vi "Process.vi"(8 "error in":errorcluster, 11 "RemoteControl":refnum<class "RemoteControl.lvclass">) -> (0 "error out":errorcluster, 3 "RemoteControl out":refnum<class "RemoteControl.lvclass">)   [LabVIEW 2016, in "RemoteControl.lvclass"]
doc: "---------------------------------------------------------------\nJKI State Machine Objects™\nhttp://jki.net/state-machine-objects/\nCopyright (C) 2005-2015, JKI <info@jki.net>\nALL RIGHTS RESERVED"
uses:
  RemoteControl.lvclass
  C:/Program Files (x86)/National Instruments/LabVIEW 2016/vi.lib/JKI/JKI SMO/SMO/SMO.lvclass
  <vilib>/NI/STM/SubVIs/MetaDataElement.ctl
  <vilib>/JKI/JKI SMO/SMO/Typedefs/Parent Call--Enum.ctl
  Typedefs/Remote-SMO-Commands-Enum.ctl
  Typedefs/PrivateEvents--RemoteControl.setAllowedRemoteAddress.ctl
  Typedefs/PrivateEvents--RemoteControl.setResults.ctl
  Typedefs/PrivateEvents--RemoteControl.setAO.ctl
  Typedefs/PrivateEvents--RemoteControl.setAI.ctl
  Typedefs/PrivateEvents--RemoteControl.setTrigger.ctl
  Typedefs/REF-cluster.ctl
  Typedefs/REF_f-array.ctl
  Typedefs/REF_phi-array.ctl
  Typedefs/AO-cluster.ctl
  Typedefs/AO_Amp-array.ctl
  Typedefs/AO_DC-array.ctl
  Typedefs/AO_f-array.ctl
  Typedefs/AO_phi-array.ctl
  Typedefs/Function-array.ctl
  Typedefs/Function-enum.ctl
  Typedefs/PrivateEvents--RemoteControl.setIVmode.ctl
  RemoteControl.lvclass/RemoteControl.ctl
  <vilib>/NI/STM/TCP/TCP Read Options.ctl
  Typedefs/PublicEvents--RemoteControl.configAO.ctl
  Typedefs/PublicEvents--RemoteControl.configREF.ctl
  Typedefs/PublicEvents--RemoteControl.configIVmode.ctl
  Typedefs/PublicEvents--RemoteControl.configRemote.ctl
  Typedefs/PublicEvents--RemoteControl.configReset.ctl
  Typedefs/PublicEvents--RemoteControl.assertTrigger.ctl
  <vilib>/NI/STM/TCP/Write Meta Data (TCP Ref).vi
  <vilib>/NI/STM/TCP/Get Connection Reference (TCP).vi
  <userlib>/_OpenG.lib/error/error.llb/Filter Error Codes (Array)__ogtk.vi
  <vilib>/NI/STM/TCP/Write Meta Data (TCP Clst).vi
  <vilib>/NI/STM/TCP/Read Message (TCP).vi
  <vilib>/NI/STM/TCP/Write Message (TCP).vi
  <vilib>/JKI/JKI SMO/SMO/SMO.lvclass
  <vilib>/NI/STM/NI STM.lvlib
  <vilib>/addons/_JKI.lib/Serialization/JSON/JKI JSON Serialization.lvlib
panel:
  out "states":string
  out "commands":string
  out "data string":string
  out "command":T1
  # "For instructions on how to use the JKI State Machine Objects, examples and video tutorials, visit:\nhttp://jki.net/state-machine-objects/\n\nJKI State Machine Objects™\nhttp://jki.net/state-machine-objects/\nCopyright (C) 2005-2015, JKI <info@jki.net>\nALL RIGHTS RESERVED"
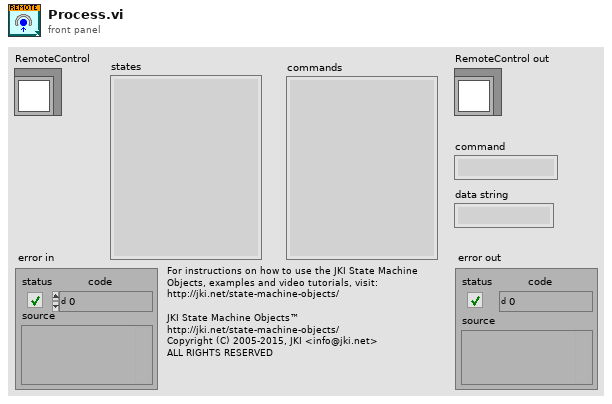
[diagram p1: front panel]
types:
  T1 = typedef "NI STM.lvlib/MetaDataElement.ctl" = string
  T2 = typedef "RemoteControl.lvclass/Remote-SMO-Commands-Enum.ctl" = enum16{"configAO", "configREF", "configIVmode", "configRemote", "configReset", "assertTrigger", "getAO", "getAI", "getResults", "getTrigger", "getIVmode", "getAOconfig", "getREFconfig", "ACK", "UNK", "CLOSE"}
  T3 = typedef "SMO.lvclass/Parent Call--Enum.ctl" = enum16{"Allows parent to run", "Does not request parent to run"}
  T4 = enum32{"invalid app kind", "Development System", "Run Time System", "Student Edition", "Embedded LabVIEW", "Evaluation", "Custom"}
  T5 = enum32{"Invalid", "Standard", "Closed", "Hidden", "Minimized", "Maximized"}
  T6 = enum32{"Bad", "Idle", "Run top level", "Running"}
  T7 = typedef "NI STM.lvlib/TCP Read Options.ctl" = cluster{"ignore timeout error":bool, "timeout ms (1000)":i32}
  T8 = typedef "RemoteControl.lvclass/PrivateEvents--RemoteControl.setAllowedRemoteAddress.ctl" = string
  T9 = typedef "NI STM.lvlib/TCP Connection Info.ctl" = cluster{"connection ID":refnum<k5>, "meta data":T1[]}
  T10 = typedef "RemoteControl.lvclass/PrivateEvents--RemoteControl.setAO.ctl" = waveform(dbl)[]
  T11 = typedef "RemoteControl.lvclass/PrivateEvents--RemoteControl.setAI.ctl" = waveform(dbl)[]
  T12 = typedef "RemoteControl.lvclass/PrivateEvents--RemoteControl.setResults.ctl" = dbl[][]
  T13 = typedef "RemoteControl.lvclass/PrivateEvents--RemoteControl.setTrigger.ctl" = bool
  T14 = typedef "AO-cluster.ctl" = cluster{"AO amp (V)":T15, "AO DC (V)":T16, "AO f (Hz)":T17, "AO phi (deg)":T18, "function":T19}
  T15 = typedef "AO_Amp-array.ctl" = dbl[]
  T16 = typedef "AO_DC-array.ctl" = dbl[]
  T17 = typedef "AO_f-array.ctl" = dbl[]
  T18 = typedef "AO_phi-array.ctl" = dbl[]
  T19 = typedef "Function-array.ctl" = T20[]
  T20 = typedef "Function-enum.ctl" = enum16{"Sine Wave", "Triangle Wave", "Square Wave", "Sawtooth Wave"}
  T21 = typedef "REF-cluster.ctl" = cluster{"REF f (Hz)":T22, "REF phi (deg)":T23}
  T22 = typedef "REF_f-array.ctl" = dbl[]
  T23 = typedef "REF_phi-array.ctl" = dbl[]
  T24 = typedef "RemoteControl.lvclass/PrivateEvents--RemoteControl.setIVmode.ctl" = bool
  T25 = cluster{"Core":cluster{"Current VI Reference":refnum<vi>, "Close Panel on Exit?":bool, "error":errorcluster}, "Self Reference":refnum<class "RemoteControl.lvclass">, "STP info":cluster{"address":string, "port":u16, "STP connection info":T9}, "remote address":string, "remote port":u16, "data string":string, "command":T1, "AllowedRemoteAddress":T8, "LocalAddress":string, "setAO":T10, "setAI":T11, "setResults":T12, "setTrigger":T13, "Channels: AO":T14, "Channels: Lockin":T21, "setIVmode":T24}
  T26 = cluster{"Current VI Reference":refnum<vi>, "Close Panel on Exit?":bool, "error":errorcluster}
  T27 = cluster{"address":string, "port":u16, "STP connection info":T9}
  T28 = typedef "SMO.lvclass/Protected Events.ctl" = cluster{"StopProcesses":refnum<user-event>, "AbortProcesses":refnum<user-event>, "Config Changed":refnum<user-event>, "Dependency":refnum<user-event>}
  T29 = typedef "RemoteControl.lvclass/PrivateEvents--Cluster.ctl" = cluster{"setAllowedRemoteAddress":refnum<user-event>, "setAO":refnum<user-event>, "setAI":refnum<user-event>, "setResults":refnum<user-event>, "setTrigger":refnum<user-event>, "setAOconfig":refnum<user-event>, "setREFconfig":refnum<user-event>, "setReset":refnum<user-event>, "setIVmode":refnum<user-event>}
  T30 = typedef "RemoteControl.lvclass/PublicEvents--RemoteControl.configAO.ctl" = cluster{"Channels: AO":T14}
  T31 = typedef "RemoteControl.lvclass/PublicEvents--RemoteControl.configREF.ctl" = cluster{"Channels: Lockin":T21}
  T32 = typedef "RemoteControl.lvclass/PublicEvents--RemoteControl.configIVmode.ctl" = bool
  T33 = typedef "RemoteControl.lvclass/PublicEvents--RemoteControl.configRemote.ctl" = bool
  T34 = typedef "RemoteControl.lvclass/PublicEvents--RemoteControl.configReset.ctl" = bool
  T35 = typedef "RemoteControl.lvclass/PublicEvents--RemoteControl.assertTrigger.ctl" = bool
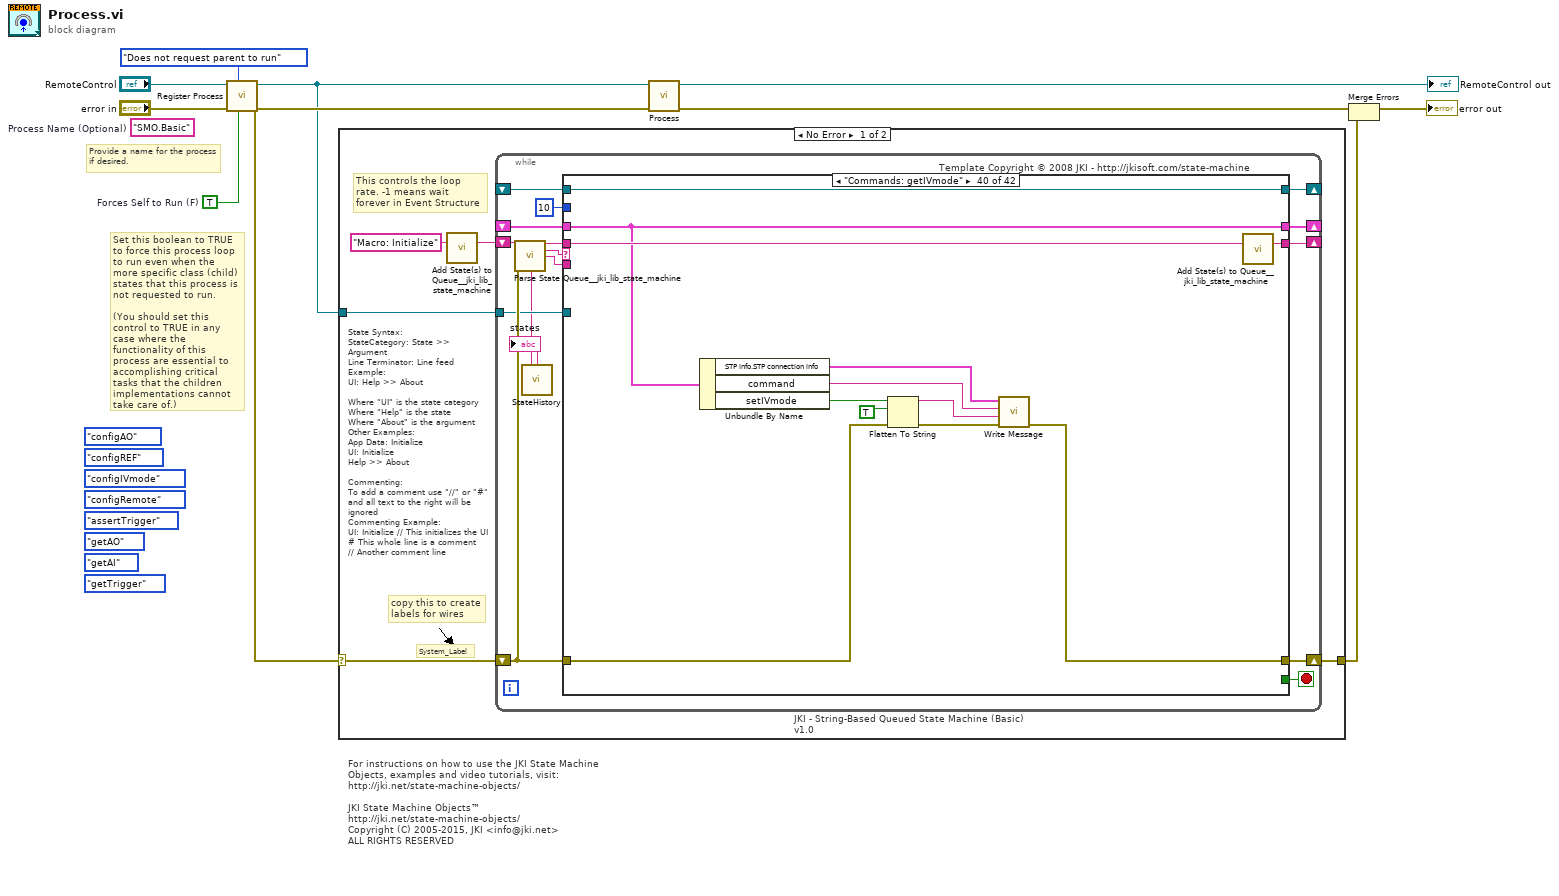
[diagram p0: block diagram]
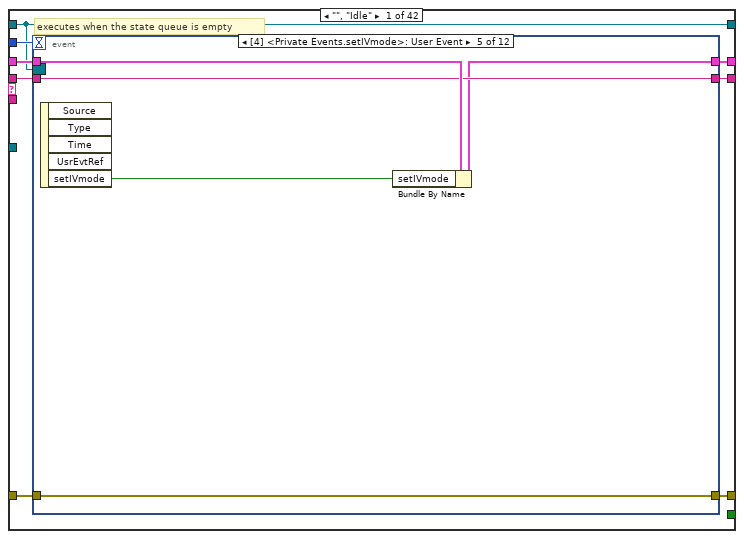
[diagram p2: hidden frame]
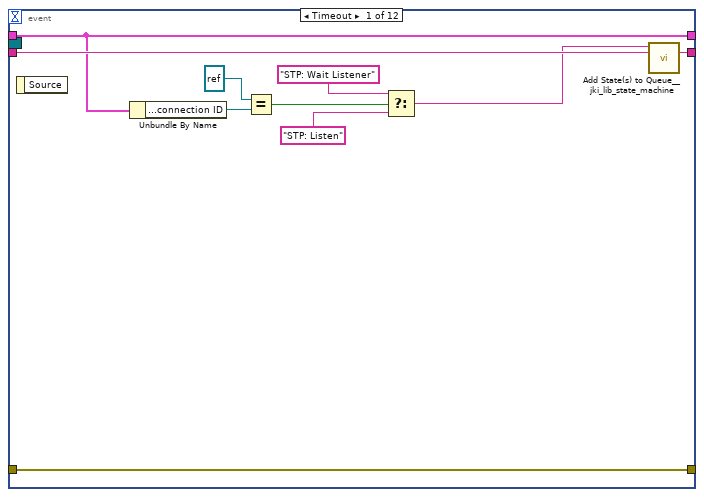
[diagram p3: hidden frame]
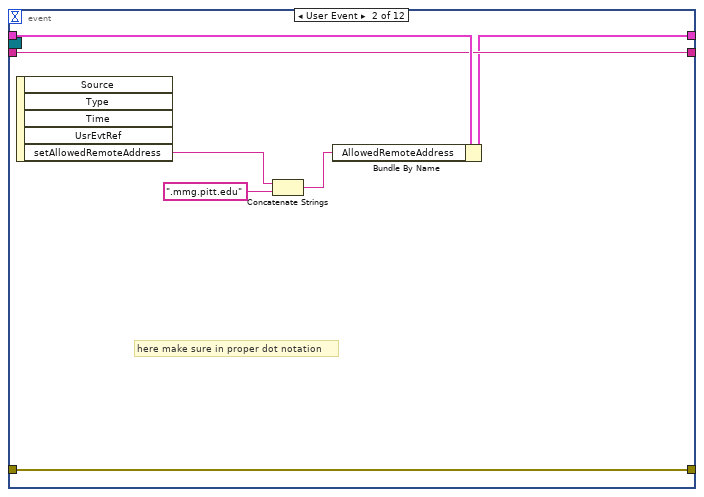
[diagram p4: hidden frame]
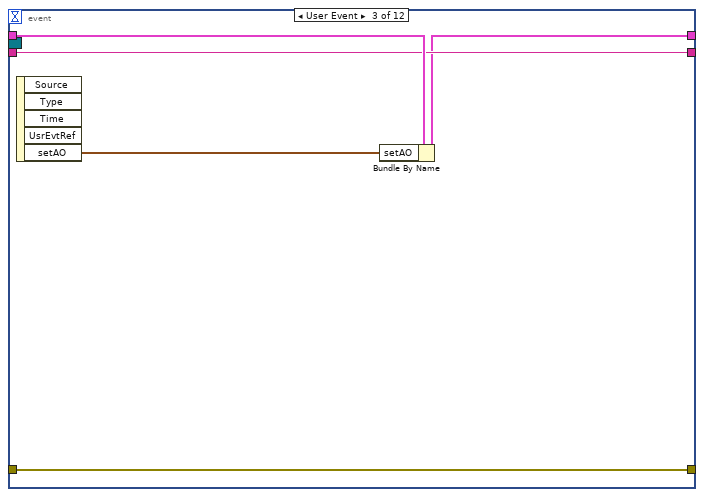
[diagram p5: hidden frame]
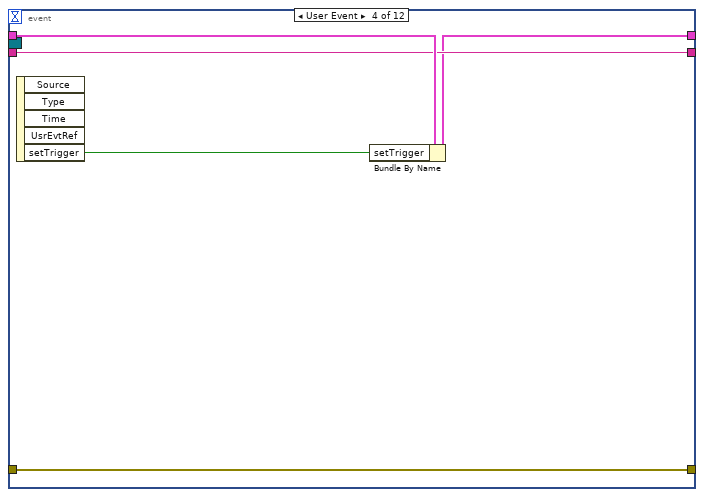
[diagram p6: hidden frame]
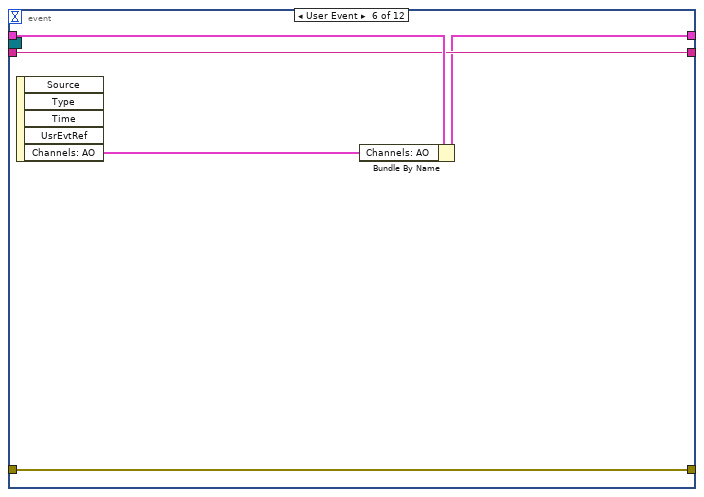
[diagram p7: hidden frame]
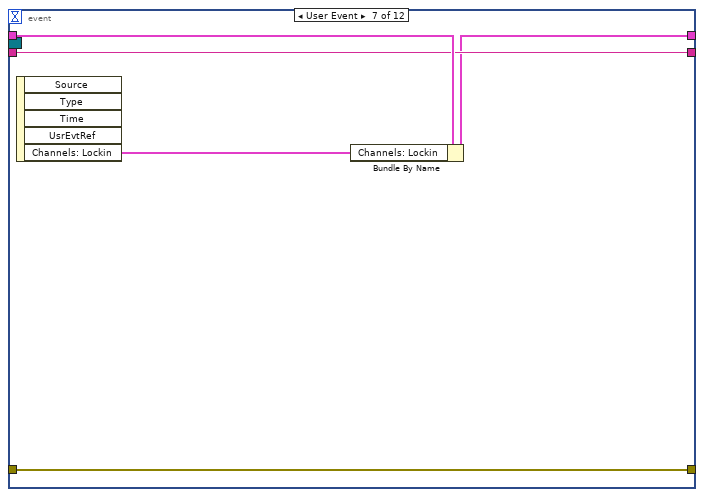
[diagram p8: hidden frame]
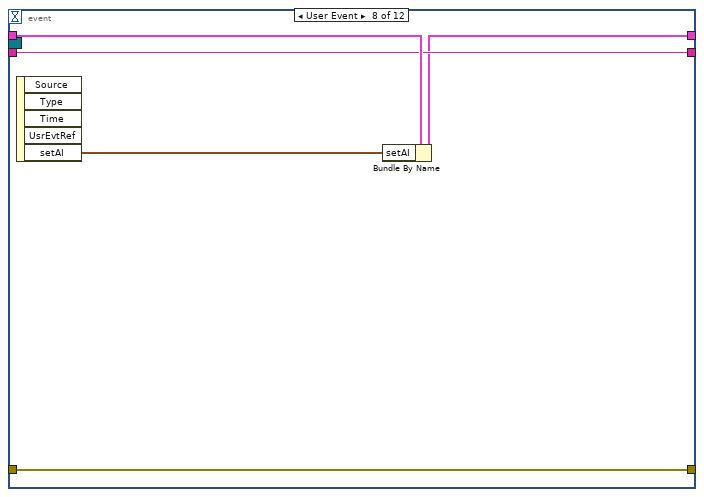
[diagram p9: hidden frame]
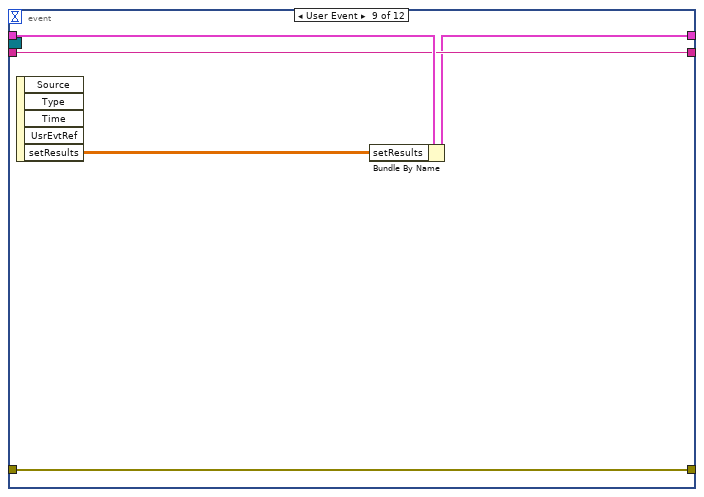
[diagram p10: hidden frame]
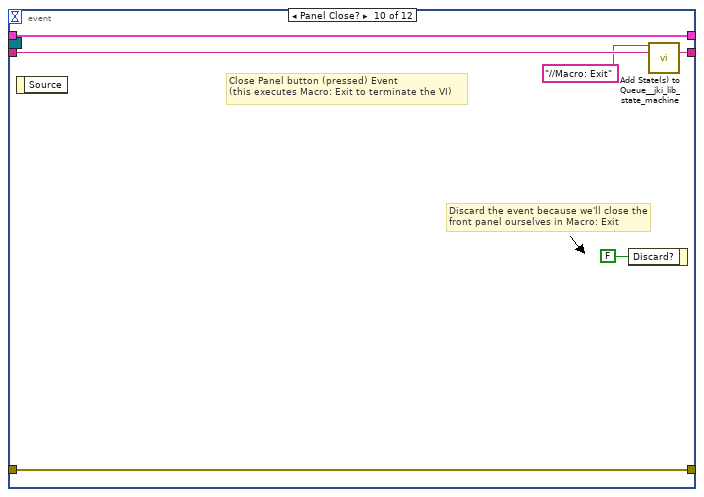
[diagram p11: hidden frame]
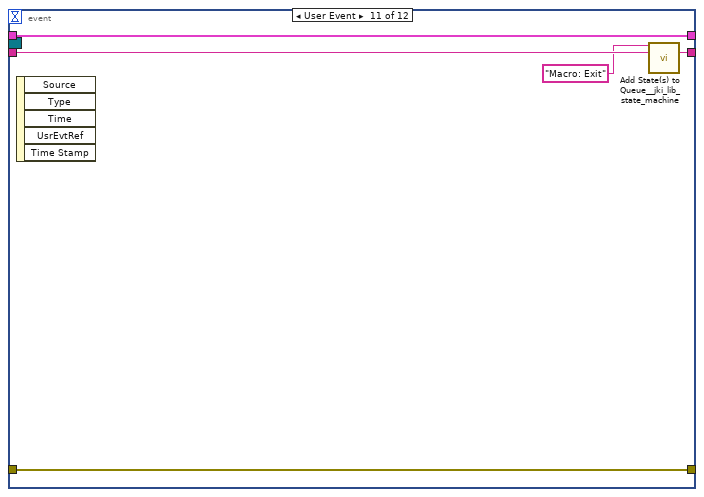
[diagram p12: hidden frame]
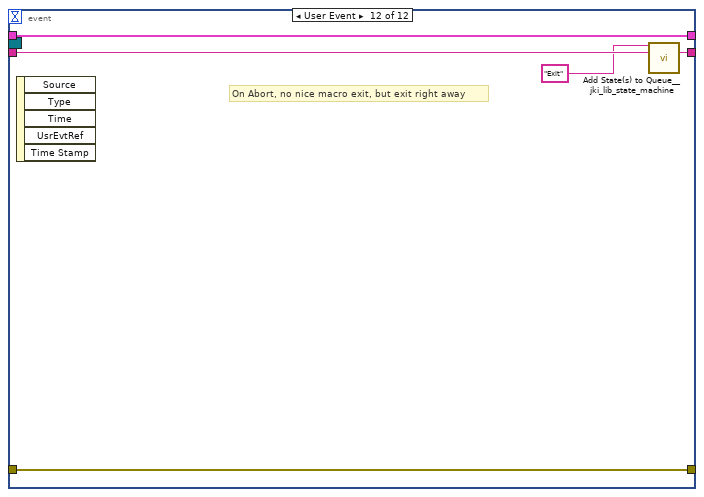
[diagram p13: hidden frame]
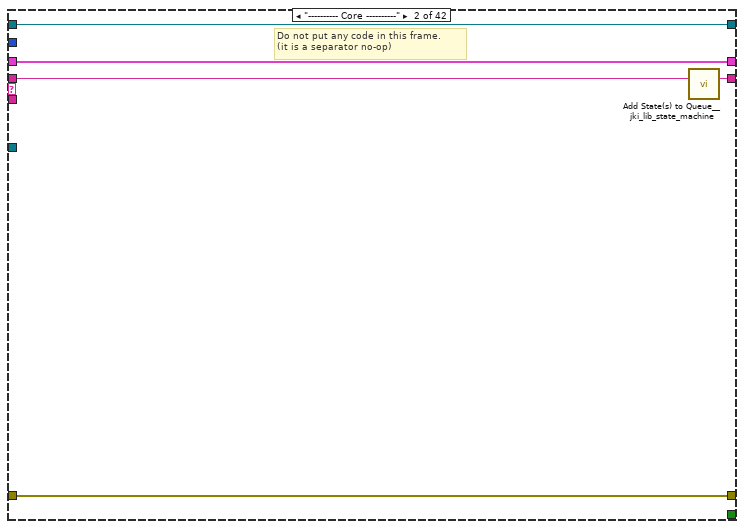
[diagram p14: hidden frame]
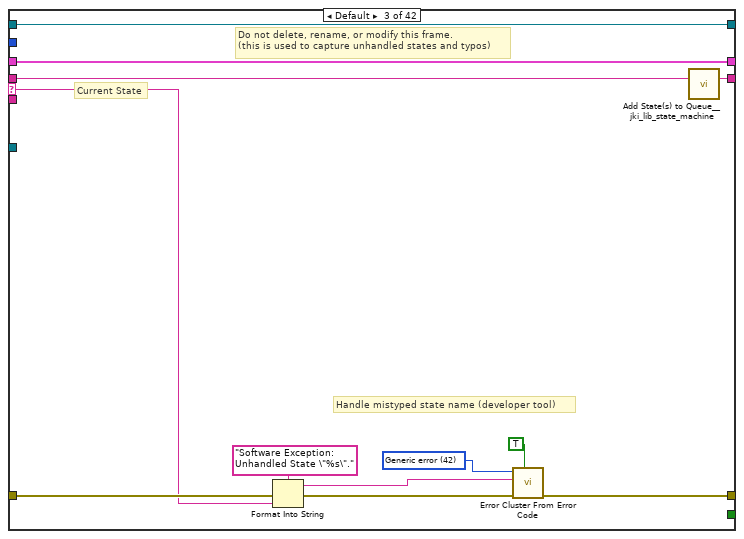
[diagram p15: hidden frame]
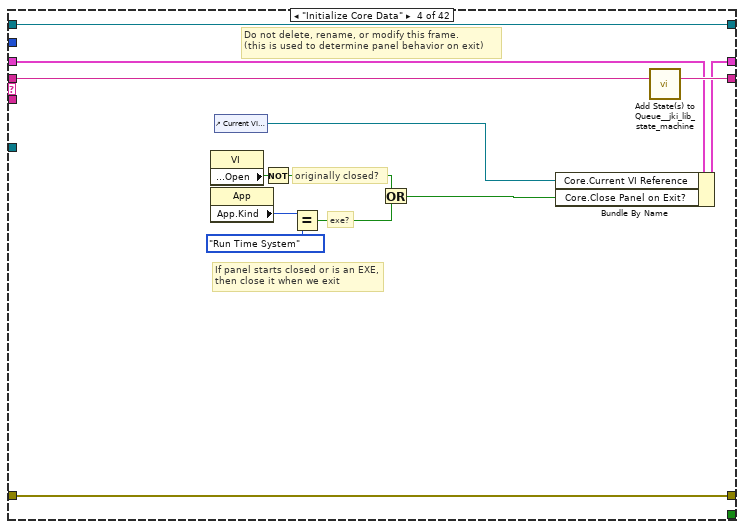
[diagram p16: hidden frame]
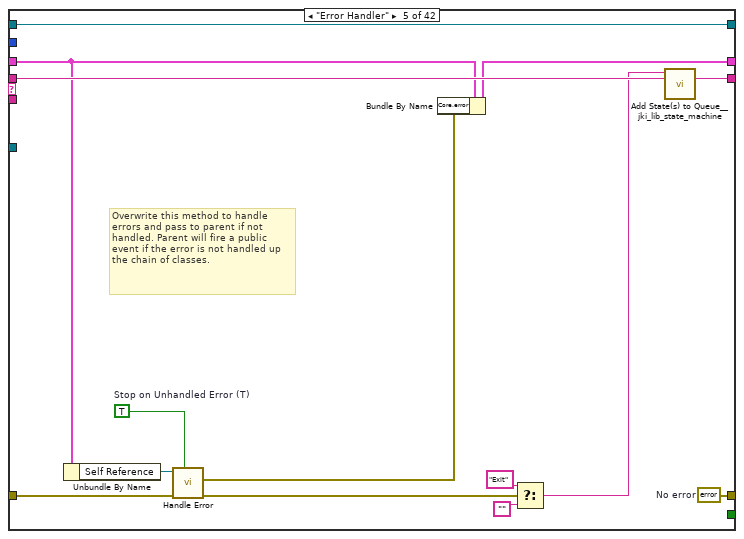
[diagram p17: hidden frame]
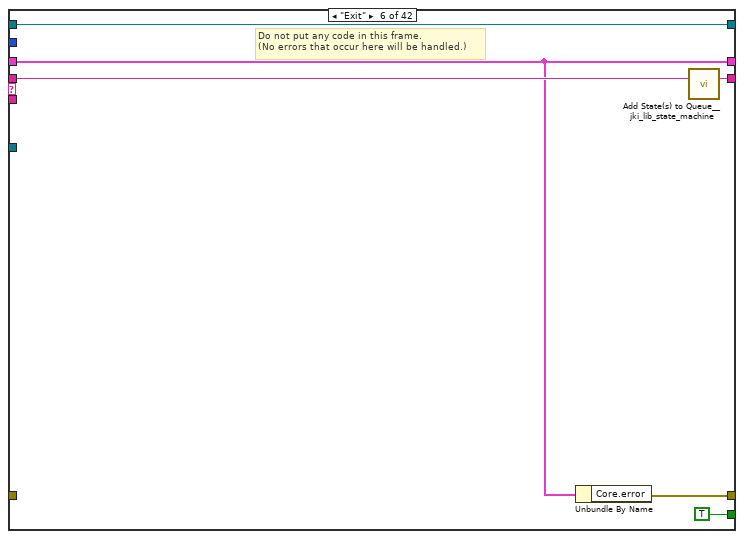
[diagram p18: hidden frame]
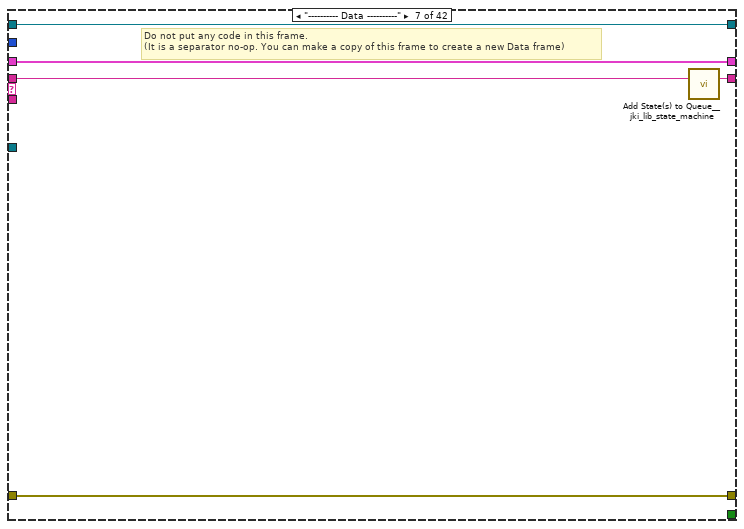
[diagram p19: hidden frame]
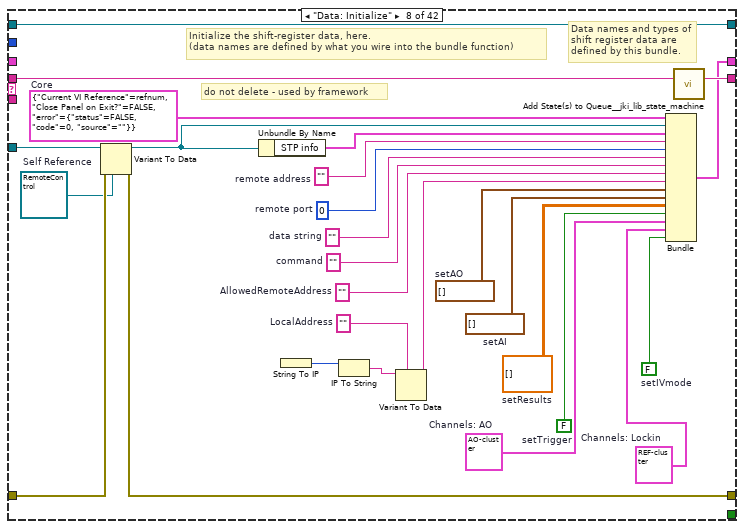
[diagram p20: hidden frame]
diagram:
  (unwired) Remote-SMO-Commands-Enum."getTrigger" ("Enum")
  (unwired) Remote-SMO-Commands-Enum."getAI" ("Enum")
  (unwired) Remote-SMO-Commands-Enum."getAO" ("Enum")
  (unwired) Remote-SMO-Commands-Enum."assertTrigger" ("Enum")
  (unwired) Remote-SMO-Commands-Enum."configRemote" ("Enum")
  (unwired) Remote-SMO-Commands-Enum."configIVmode" ("Enum")
  (unwired) Remote-SMO-Commands-Enum."configREF" ("Enum")
  (unwired) Remote-SMO-Commands-Enum."configAO" ("Enum")
  w1 = TRUE  # Forces Self to Run (F)
  (unwired) "SMO.Basic"  # Process Name (Optional)
  # "Provide a name for the process\nif desired."
  # "Set this boolean to TRUE to force this process loop to run even when the more specific class (child) states that this process is not requested to run.\n\n(You should set this control to TRUE in any case where the functionality of this process are essential to accomplishing critical tasks that the children implementations cannot take care of.)"
  # "For instructions on how to use the JKI State Machine Objects, examples and video tutorials, visit:\nhttp://jki.net/state-machine-objects/\n\nJKI State Machine Objects™\nhttp://jki.net/state-machine-objects/\nCopyright (C) 2005-2015, JKI <info@jki.net>\nALL RIGHTS RESERVED"
  n1 = call <vilib>:"Register Process.vi"("Forces Self to Run (F)"=w1, "Parent Call"=Parent_Call--Enum."Does not request parent to run", "error in (no error)"="error in", "SMO"="RemoteControl") -> ("error out"=w7:errorcluster, "SMO out"=w6:refnum<class "RemoteControl.lvclass">)  [unwired: 6 in]
  n2 = case shown="No Error" w7 {
    selector: w7 -> [w12 w652]
    tunnel: w6 -> [w13 _]
    tunnel: [w11 w652] -> w3
    frame No Error {
      # "State Syntax:\nStateCategory: State >> Argument\nLine Terminator: Line feed\nExample:\nUI: Help >> About\n\nWhere \"UI\" is the state category\nWhere \"Help\" is the state\nWhere \"About\" is the argument\nOther Examples:\nApp Data: Initialize\nUI: Initialize\nHelp >> About\n\nCommenting:\nTo add a comment use \"//\" or \"#\" and all text to the right will be ignored\nCommenting Example:\nUI: Initialize // This initializes the UI\n# This whole line is a comment\n// Another comment line"
      # "copy this to create labels for wires"
      # "This controls the loop rate. -1 means wait forever in Event Structure"
      # "System_Label"
      n3 = call <vilib>:"Add State(s) to Queue__jki_lib_state_machine.vi"("State(s) in (\"\")"="Macro: Initialize") -> ("States Out"=w15:string)  [unwired: 14 in]
      n4 = while "JKI - String-Based Queued State Machine (Basic) v1.0" {
        shift-right: [w24] -> _
        shift-left: _ -> [w23]
        shift-right: [w27] -> w11
        shift-left: w12 -> [w21]
        shift-right: [w26] -> _
        shift-left: w15 -> [w17]
        tunnel: w13 -> [w20]
        shift-right: [w19] -> _
        shift-left: _ -> [w18]
        stop <- w25 stop-if-true
        # "Template Copyright © 2008 JKI - http://jkisoft.com/state-machine"
        n5 = call <vilib>:"Parse State Queue__jki_lib_state_machine.vi"("State Queue"=w17, "Error In (no error)"=w21) -> ("Remaining States"=w29:string, "Current State"=w30:string, "Arguments"=w28:string)  [unwired: 11 in]
        n6 = call "StateHistory.vi"("Current State in"=w17) -> ("delimited string"=→"states":string)  [unwired: 9 in, 1 out]
        n7 = case shown="\"Commands: getIVmode\"" w30 {
          selector: w30 -> [_ _ w113 _ _ _ _ _ _ _ _ _ _ _ _ _ _ _ _ _ _ _ _ _ _ _ _ _ _ _ _ _ _ _ _ _ _ _ _ _ _ _]
          tunnel: w29 -> [w38 w111 w117 w136 w150 w156 w161 w188 w195 w200 w205 w212 w228 w260 w274 w288 w293 w304 w309 w322 w328 w333 w353 w391 w408 w450 w468 w480 w485 w500 w515 w528 w541 w554 w567 w579 w591 w603 w615 w627 w639 w651]
          tunnel: w28 -> [_ _ _ _ _ _ _ _ _ _ _ w206 w222 _ _ _ _ _ _ _ _ _ _ _ _ _ _ _ _ _ _ _ _ _ _ _ _ _ _ _ _ _]
          tunnel: w23 -> [w36 w108 w115 w127 w144 w152 w158 _ w190 w197 w203 w210 w224 w257 w270 w279 w290 w301 w306 w320 w326 w331 w342 w388 w405 w437 w455 w472 w483 w493 w507 w516 w537 w551 w564 w576 w587 w599 w611 w623 w635 w647]
          tunnel: [w35 w109 w119 w133 w145 w151 w159 w184 w191 w198 w202 w207 w225 w258 w272 w286 w291 w295 w307 w315 w324 w329 w348 w384 w394 w444 w462 w469 w481 w491 w505 w517 w536 w543 w555 w570 w581 w593 w605 w617 w629 w641] -> w27
          tunnel: w21 -> [w34 w109 w118 w133 w146 _ w159 w185 w192 w198 w202 w208 w226 w258 w272 w286 w291 w296 w307 w316 w324 w329 w349 w385 w402 w445 w463 w475 w481 w492 w506 w520 w533 w548 w561 w571 w582 w594 w606 w618 w630 w642]
          tunnel: [w37 w110 w116 w135 w149 w155 w160 w187 w194 w199 w204 w211 w227 w259 w273 w287 w292 w303 w308 w321 w327 w332 w352 w390 w407 w449 w467 w479 w484 w499 w514 w527 w540 w553 w566 w578 w590 w602 w614 w626 w638 w650] -> w26
          tunnel: [_ _ _ _ _ TRUE _ _ _ _ _ _ _ _ _ _ _ _ _ _ _ _ _ _ _ _ _ _ _ _ _ _ _ _ _ _ _ _ _ _ _ _] -> w25
          tunnel: [w33 w108 w115 w134 w143 w152 w158 w186 w190 w197 w203 w210 w224 w257 w270 w279 w290 w301 w306 w320 w326 w331 w347 w387 w404 w436 w454 w471 w483 w493 w507 w516 w537 w551 w564 w576 w587 w599 w611 w623 w635 w647] -> w24
          tunnel: 10 ("Timeout") -> [w32 _ _ _ _ _ _ _ _ _ _ _ _ _ _ _ _ _ _ _ _ _ _ _ _ _ _ _ _ _ _ _ _ _ _ _ _ _ _ _ _ _]
          tunnel: w20 -> [_ _ _ _ _ _ _ w182 _ _ _ _ _ _ _ _ _ _ _ _ _ _ _ _ _ _ _ _ _ _ _ _ _ _ _ _ _ _ _ _ _ _]
          tunnel: [w31 w107 w112 w124 w148 w153 w157 w181 w189 w196 w201 w209 w221 w256 w271 w280 w289 w302 w305 w319 w325 w330 w351 w389 w406 w448 w466 w478 w482 w498 w513 w526 w539 w552 w565 w577 w589 w601 w613 w625 w637 w649] -> w19
          tunnel: w18 -> [w31 w107 w112 w124 w148 w153 w157 w181 w189 w196 w201 w209 w221 w256 w271 w280 w289 w302 w305 _ w325 w330 w351 w389 w406 w448 w466 w478 w482 w498 w513 w526 w539 w552 w565 w577 w589 w601 w613 w625 w637 w649]
          frame "", "Idle" {
            # "executes when the state queue is empty"
            n8 = event shown="[4] <Private Events.setIVmode>: User Event" {
              selector: w31 -> [_ _ _ _ _ _ _ _ _ _ _ _]
              dyn-events: _ -> [_ _ _ _ _ _ _ _ _ _ _ _]
              timeout: w32 -> [_ _ _ _ _ _ _ _ _ _ _ _]
              tunnel: w38 -> [w48 w54 w59 w64 w69 w74 w79 w84 w89 w96 w101 w106]
              tunnel: [w47 w54 w59 w64 w69 w74 w79 w84 w89 w95 w100 w105] -> w37
              tunnel: w36 -> [w46 w55 w60 w65 w70 w75 w80 w85 w90 w93 w98 w103]
              tunnel: [w45 w52 w57 w62 w67 w72 w77 w82 w87 w94 w99 w104] -> w35
              tunnel: w34 -> [w45 w52 w57 w62 w67 w72 w77 w82 w87 w94 w99 w104]
              tunnel: [w46 w53 w58 w63 w68 w73 w78 w83 w88 w93 w98 w103] -> w33
              event Timeout {
                n9 = event-data() -> ()  [unwired: 1 in, 1 out]
                n10 = Unbundle By Name(w46) -> ("STP info.STP connection info.connection ID"=w44:refnum<k5>)
                n11 = Equal?(x=refnum<k5> refnum ("connection ID"), y=w44) -> (x = y?=w43:bool)
                n12 = Select(t="STP: Wait Listener" ("State(s) in Front (\"\")"), s=w43, f="STP: Listen" ("State(s) in Front (\"\")")) -> (s? t:f=w39:string)
                n13 = call <vilib>:"Add State(s) to Queue__jki_lib_state_machine.vi"("State(s) in Front (\"\")"=w39, "State(s) in (\"\")"=w48) -> ("States Out"=w47:string)  [unwired: 13 in]
              }
              event User Event {
                # "here make sure in proper dot notation"
                n14 = event-data() -> ("setAllowedRemoteAddress"=w49:T8)  [unwired: 1 in, 4 out]
                n15 = Concatenate Strings(w49, ".mmg.pitt.edu" ("string")) -> (w50:string)
                n16 = Bundle By Name(cluster=w55, "AllowedRemoteAddress"=w50) -> (w53:T25)
              }
              event User Event {
                n17 = event-data() -> ("setAO"=w56:T10)  [unwired: 1 in, 4 out]
                n18 = Bundle By Name(cluster=w60, "setAO"=w56) -> (w58:T25)
              }
              event User Event {
                n19 = event-data() -> ("setTrigger"=w61:T13)  [unwired: 1 in, 4 out]
                n20 = Bundle By Name(cluster=w65, "setTrigger"=w61) -> (w63:T25)
              }
              event User Event {
                n21 = event-data() -> ("setIVmode"=w66:T24)  [unwired: 1 in, 4 out]
                n22 = Bundle By Name(cluster=w70, "setIVmode"=w66) -> (w68:T25)
              }
              event User Event {
                n23 = event-data() -> ("Channels: AO"=w71:T14)  [unwired: 1 in, 4 out]
                n24 = Bundle By Name(cluster=w75, "Channels: AO"=w71) -> (w73:T25)
              }
              event User Event {
                n25 = event-data() -> ("Channels: Lockin"=w76:T21)  [unwired: 1 in, 4 out]
                n26 = Bundle By Name(cluster=w80, "Channels: Lockin"=w76) -> (w78:T25)
              }
              event User Event {
                n27 = event-data() -> ("setAI"=w81:T11)  [unwired: 1 in, 4 out]
                n28 = Bundle By Name(cluster=w85, "setAI"=w81) -> (w83:T25)
              }
              event User Event {
                n29 = event-data() -> ("setResults"=w86:T12)  [unwired: 1 in, 4 out]
                n30 = Bundle By Name(cluster=w90, "setResults"=w86) -> (w88:T25)
              }
              event Panel Close? {
                # "Discard the event because we'll close the front panel ourselves in Macro: Exit"
                # "Close Panel button (pressed) Event\n(this executes Macro: Exit to terminate the VI)"
                n31 = event-data() -> ()  [unwired: 1 in, 1 out]
                n32 = event-data("Discard?"=FALSE) -> ()  [unwired: 1 in, 1 out]
                n33 = call <vilib>:"Add State(s) to Queue__jki_lib_state_machine.vi"("State(s) in Front (\"\")"="//Macro: Exit", "State(s) in (\"\")"=w96) -> ("States Out"=w95:string)  [unwired: 13 in]
              }
              event User Event {
                n34 = event-data() -> ()  [unwired: 1 in, 5 out]
                n35 = call <vilib>:"Add State(s) to Queue__jki_lib_state_machine.vi"("State(s) in Front (\"\")"="Macro: Exit", "State(s) in (\"\")"=w101) -> ("States Out"=w100:string)  [unwired: 13 in]
              }
              event User Event {
                # "On Abort, no nice macro exit, but exit right away"
                n36 = event-data() -> ()  [unwired: 1 in, 5 out]
                n37 = call <vilib>:"Add State(s) to Queue__jki_lib_state_machine.vi"("State(s) in Front (\"\")"="Exit", "State(s) in (\"\")"=w106) -> ("States Out"=w105:string)  [unwired: 13 in]
              }
            }
          }
          frame "---------- Core ----------" {
            # "Do not put any code in this frame.\n(it is a separator no-op)"
            n38 = call <vilib>:"Add State(s) to Queue__jki_lib_state_machine.vi"("State(s) in (\"\")"=w111) -> ("States Out"=w110:string)  [unwired: 14 in]
          }
          frame Default {
            w122 = 42 items=["No error", "Argument error", "Memory is full", "Out of zone", "End of file", "File already open", "Generic file I/O error", "File not found", "File permission error", "Disk is full", "Duplicate path", "Too many files open", "System feature not enabled", "Resource file not found", "Cannot add resource", "Resource not found", "Image not found", "Image memory error", "Pen does not exist", "Config type invalid", "Config token not found", "Config parse error", "Config memory error", "Bad external code format", "Bad external code offset", "External code not present", "Null window", "Destroy window error", "Null menu", "Print aborted", "Bad print record", "Print driver error", "Windows error during printing", "Memory error during printing", "Print dialog error", "Generic print error", "Invalid device refnum", "Device not found", "Device parameter error", "Device unit error", "Cannot open device", "Device call aborted", "Generic error", "Cancelled by user", "Object ID too low", "Object ID too high", "Object not in heap", "Unknown heap", "Unknown object (invalid DefProc)", "Unknown object (DefProc not in table)", "Message out of range", "Invalid (null) method", "Unknown message", "Manager call not supported", "Bad address", "Network operation in progress", "Network operation timed out", "Connection is busy", "Network attribute not supported", "Network error", "Address in use", "System out of memory", "Connection aborted", "Connection refused", "Not connected", "Already connected", "Connection closed", "Initialization error (interapplication manager)", "Bad occurrence", "Wait on unbound occurrence handler", "Occurrence queue overflow", "Datalog type conflict", "Unused", "Unrecognized type (interapplication manager)", "Memory corrupt", "Failed to make temporary DLL", "Old CIN version", "Drag socket not found", "Failed to load drop-object", "Failed to register OLE object", "Failed to release OLE object", "Format specifier type mismatch", "Unknown format specifier", "Too few format specifiers", "Too many format specifiers", "Scan failed", "Newer CIN version", "Error converting to variant", "Runtime menu error", "Password tampered", "Variant attribute not found", "Incompatible variant data type", "Event data is not available", "Event Store is not present", "Occurrence is not found", "Event Queue is not created", "Event info is not available", "Refnum passed is NULL", "Error retrieving Class GUID", "Error retrieving CoClass GUID", "Error retrieving TypeLib GUID.", "Bad built application magic bytes.", "Specific driver is different from the specific driver associated with the Logical Name.", "There is no session opened to the class driver.", "Max Error", "MAX - Error with config objects", "MAX - Error loading configuration", "MAX - Group not supported"]
            # "Current State"
            # "Do not delete, rename, or modify this frame.\n(this is used to capture unhandled states and typos)"
            # "Handle mistyped state name (developer tool)"
            n39 = Format Into String(format string="Software Exception: Unhandled State \"%s\"." ("message"), error in=w118, w113) -> (resulting string=w121:string, error out=w120:errorcluster)  [unwired: 1 in]
            n40 = call <vilib>:"Error Cluster From Error Code.vi"("show call chain? (False)"=TRUE, "error in (no error)"=w120, "error message (\"\")"=w121, "error code (0)"=w122) -> ("error out"=w119:errorcluster)  [unwired: 5 in]
            n41 = call <vilib>:"Add State(s) to Queue__jki_lib_state_machine.vi"("State(s) in (\"\")"=w117) -> ("States Out"=w116:string)  [unwired: 14 in]
          }
          frame "Initialize Core Data" {
            # "Do not delete, rename, or modify this frame.\n(this is used to determine panel behavior on exit)"
            # "originally closed?"
            # "exe?"
            # "If panel starts closed or is an EXE, then close it when we exit"
            n42 = property class="VI"() -> ("Front Panel.Open"=w132:bool)  [unwired: 2 in, 2 out]
            n43 = property class="App"() -> ("App.Kind"=w131:T4)  [unwired: 2 in, 2 out]
            n44 = control-ref of="Current VI Reference"() -> (w125:refnum<vi>)
            n45 = Not(x=w132) -> (.not. x?=w129:bool)
            n46 = Equal?(x=w131, y=T4."Run Time System" ("Application:Kind")) -> (x = y?=w128:bool)
            n47 = Or(x=w129, y=w128) -> (x .or. y?=w126:bool)
            n48 = Bundle By Name(cluster=w127, "Core.Current VI Reference"=w125, "Core.Close Panel on Exit?"=w126) -> (w134:T25)
            n49 = call <vilib>:"Add State(s) to Queue__jki_lib_state_machine.vi"("State(s) in (\"\")"=w136) -> ("States Out"=w135:string)  [unwired: 14 in]
          }
          frame "Error Handler" {
            w137 = TRUE  # Stop on Unhandled Error (T)
            w145 = errorcluster {"status"=FALSE, "code"=0, "source"=""}  # No error
            # "Overwrite this method to handle errors and pass to parent if not handled. Parent will fire a public event if the error is not handled up the chain of classes."
            n50 = Unbundle By Name(w144) -> ("Self Reference"=w147:refnum<class "RemoteControl.lvclass">)
            n51 = call-dynamic "Handle Error.vi"("Stop on Unhandled Error (T)"=w137, "error in"=w146, "SMO"=w147) -> ("handling error"=w138:errorcluster, "Unhandled error"=w141:errorcluster)  [unwired: 6 in, 1 out]
            n52 = Bundle By Name(cluster=w144, "Core.error"=w141) -> (w143:T25)
            n53 = Select(t="Exit", s=w138, f="") -> (s? t:f=w142:string)
            n54 = call <vilib>:"Add State(s) to Queue__jki_lib_state_machine.vi"("State(s) in Front (\"\")"=w142, "State(s) in (\"\")"=w150) -> ("States Out"=w149:string)  [unwired: 13 in]
          }
          frame "Exit" {
            # "Do not put any code in this frame.\n(No errors that occur here will be handled.)"
            n55 = Unbundle By Name(w152) -> ("Core.error"=w151:errorcluster)
            n56 = call <vilib>:"Add State(s) to Queue__jki_lib_state_machine.vi"("State(s) in (\"\")"=w156) -> ("States Out"=w155:string)  [unwired: 14 in]
          }
          frame "---------- Data ----------" {
            # "Do not put any code in this frame.\n(It is a separator no-op. You can make a copy of this frame to create a new Data frame)"
            n57 = call <vilib>:"Add State(s) to Queue__jki_lib_state_machine.vi"("State(s) in (\"\")"=w161) -> ("States Out"=w160:string)  [unwired: 14 in]
          }
          frame "Data: Initialize" {
            w162 = T24 FALSE  # setIVmode
            w163 = T14 {"AO amp (V)"=[0.01, 0.0, 0.0, 0.0, 0.0, 0.0, 0.0, 0.0], "AO DC (V)"=[0.0, 0.0, 0.0, 0.0, 0.0, 0.0, 0.0, 0.0], "AO f (Hz)"=[13.1, 13.0, 13.0, 13.0, 13.0, 13.0, 13.0, 13.0], "AO phi (deg)"=[0.0, 0.0, 0.0, 0.0, 0.0, 0.0, 0.0, 0.0], "function"=[enum."Sine Wave", enum."Sine Wave", enum."Sine Wave", enum."Sine Wave", enum."Sine Wave", enum."Sine Wave", enum."Sine Wave", enum."Sine Wave"]}  # Channels: AO
            w168 = T21 {"REF f (Hz)"=[13.0], "REF phi (deg)"=[0.0, 0.0, 0.0, 0.0, 0.0, 0.0, 0.0, 0.0]}  # Channels: Lockin
            w164 = T13 FALSE  # setTrigger
            w166 = T11 []  # setAI
            w167 = T10 []  # setAO
            w165 = T12 []  # setResults
            w170 = ""  # LocalAddress
            w173 = T8 ""  # AllowedRemoteAddress
            w174 = T1 ""  # command
            w175 = ""  # data string
            w177 = u16 0  # remote port
            w180 = T26 {"Current VI Reference"=refnum, "Close Panel on Exit?"=FALSE, "error"={"status"=FALSE, "code"=0, "source"=""}}  # Core
            w183 = refnum<class "RemoteControl.lvclass"> refnum  # Self Reference
            w176 = ""  # remote address
            # "do not delete - used by framework"
            # "Data names and types of shift register data are defined by this bundle."
            # "Initialize the shift-register data, here.\n(data names are defined by what you wire into the bundle function)"
            n58 = Variant To Data(error in=w185, type=w183, Variant=w182) -> (data=w179:refnum<class "RemoteControl.lvclass">, error out=w184:errorcluster)
            n59 = Unbundle By Name(w179) -> ("STP info"=w178:T27)
            n60 = String To IP() -> (0:w172:u32)  [unwired: 1 in]
            n61 = IP To String(2:w172) -> (0:w171:string)  [unwired: 1 in]
            n62 = Variant To Data(type=w170, Variant=w171) -> (data=w169:string)  [unwired: 1 in, 1 out]
            n63 = Bundle("Core"=w180, "Self Reference"=w179, "STP info"=w178, "remote address"=w176, "remote port"=w177, "data string"=w175, "command"=w174, "AllowedRemoteAddress"=w173, "LocalAddress"=w169, "setAO"=w167, "setAI"=w166, "setResults"=w165, "setTrigger"=w164, "Channels: AO"=w163, "Channels: Lockin"=w168, "setIVmode"=w162) -> (w186:T25)  [unwired: 1 in]
            n64 = call <vilib>:"Add State(s) to Queue__jki_lib_state_machine.vi"("State(s) in (\"\")"=w188) -> ("States Out"=w187:string)  [unwired: 14 in]
          }
          frame "Data: Cleanup" {
            # "Cleanup any data and references, here.\n(this is called automatically, by the Macro: Exit)"
            n65 = Unbundle By Name(w190) -> ("Core.Current VI Reference"=w193:refnum<vi>)
            n66 = Close Reference(reference=w193, error in (no error)=w192) -> (error out=w191:errorcluster)
            n67 = call <vilib>:"Add State(s) to Queue__jki_lib_state_machine.vi"("State(s) in (\"\")"=w195) -> ("States Out"=w194:string)  [unwired: 14 in]
          }
          frame "---------- UI ----------" {
            # "Do not put any code in this frame.\n(It is a separator no-op. You can make a copy of this frame to create a new UI frame)"
            n68 = call <vilib>:"Add State(s) to Queue__jki_lib_state_machine.vi"("State(s) in (\"\")"=w200) -> ("States Out"=w199:string)  [unwired: 14 in]
          }
          frame "UI: Initialize" {
            # "Initialize the User Interface, here.\n(this is called automatically, by the Macro: Init)"
            n69 = call <vilib>:"Add State(s) to Queue__jki_lib_state_machine.vi"("State(s) in (\"\")"=w205) -> ("States Out"=w204:string)  [unwired: 14 in]
          }
          frame "UI: Cursor Set" {
            # "Argument"
            # "Initialize the User Interface, here.\n(this is called automatically, by the Macro: Init)"
            n70 = disable-structure shown="Default" {
              disable-tunnel: w208 -> [w213 w216]
              disable-tunnel: [w213 w215] -> w207
              disable-tunnel: w206 -> [_ w214]
              frame condition #0 {
              }
              frame condition #1 (active) {
                n71 = case shown="\"Idle\", Default" w214 {
                  tunnel: w216 -> [w218 w220]
                  tunnel: [w217 w219] -> w215
                  frame "Idle", Default {
                    n72 = call <vilib>:"Unset Busy.vi"("error in (no error)"=w218) -> ("error out"=w217:errorcluster)  [unwired: 10 in]
                  }
                  frame "Busy" {
                    n73 = call <vilib>:"Set Busy.vi"("error in (no error)"=w220) -> ("error out"=w219:errorcluster)  [unwired: 9 in, 1 out]
                  }
                }
              }
            }
            n74 = call <vilib>:"Add State(s) to Queue__jki_lib_state_machine.vi"("State(s) in (\"\")"=w212) -> ("States Out"=w211:string)  [unwired: 14 in]
          }
          frame "UI: Front Panel State" {
            # "Argument"
            # "Set Front Panel Open or Closed\n(Usage: \"UI: Front Panel State >> Open|Close\")"
            n75 = Unbundle By Name(w224) -> ("Core.Current VI Reference"=w223:refnum<vi>)
            n76 = disable-structure shown="Default" {
              disable-tunnel: w226 -> [w232 w255]
              disable-tunnel: [w231 w255] -> w225
              disable-tunnel: w223 -> [w230 _]
              disable-tunnel: w222 -> [w229 _]
              frame condition #0 (active) {
                n77 = case shown="\"Close\"" w229 {
                  tunnel: w232 -> [w236 w249]
                  tunnel: [w238 w250] -> w231
                  tunnel: w230 -> [w237 w247]
                  frame "Open", Default {
                    n78 = property class="VI"(reference=w237, error in=w236) -> (reference out=w234:refnum<vi>, error out=w235:errorcluster, "FP.State"=w233:T5)
                    n79 = case shown="\"Closed\"" w233 {
                      tunnel: [w241 w244] -> w238
                      tunnel: w235 -> [w240 w244]
                      tunnel: w234 -> [w239 _]
                      frame "Closed" {
                        n80 = invoke class="VI" method="FP.Open"(reference=w239, error in=w240, "Activate"=TRUE, "State"=T5."Standard") -> (error out=w241:errorcluster)  [unwired: 1 in, 4 out]
                      }
                      frame Default {
                      }
                    }
                  }
                  frame "Close" {
                    n81 = property class="VI"(reference=w247, error in=w249) -> (reference out=w246:refnum<vi>, error out=w248:errorcluster, "FP.State"=w245:T5)
                    n82 = case shown="Default" w245 {
                      tunnel: [w251 w254] -> w250
                      tunnel: w248 -> [w251 w253]
                      tunnel: w246 -> [_ w252]
                      frame "Invalid", "Closed" {
                      }
                      frame Default {
                        n83 = invoke class="VI" method="FP.Close"(reference=w252, error in=w253) -> (error out=w254:errorcluster)  [unwired: 1 in, 2 out]
                      }
                    }
                  }
                }
              }
              frame condition #1 {
              }
            }
            n84 = call <vilib>:"Add State(s) to Queue__jki_lib_state_machine.vi"("State(s) in (\"\")"=w228) -> ("States Out"=w227:string)  [unwired: 14 in]
          }
          frame "---------- Macro ----------" {
            # "Do not put any code in this frame.\n(It is a separator no-op. You can make a copy of this frame to create a new Macro frame)"
            n85 = call <vilib>:"Add State(s) to Queue__jki_lib_state_machine.vi"("State(s) in (\"\")"=w260) -> ("States Out"=w259:string)  [unwired: 14 in]
          }
          frame "Macro: Initialize" {
            w265 = "UI: Initialize\nUI: Front Panel State >> Open"  # UI: Initialize UI: Front Panel State >> Open
            w261 = "Process: Sync"
            # "Initialization Macro\n(This is called once, when the VI starts)"
            n86 = control-ref of="This VI"() -> (w263:refnum<vi>)
            n87 = property class="VI"(reference=w263) -> ("Exec.State"=w262:T6)  [unwired: 1 in, 2 out]
            n88 = Equal?(x=w262, y=T6."Run top level") -> (x = y?=w268:bool)
            n89 = Select(t=w261, s=w268, f="") -> ()  [unwired: 1 out]
            n90 = call <vilib>:"Add State(s) to Queue__jki_lib_state_machine.vi"("State(s) in Front (\"\")"="Data: Initialize\nInitialize Core Data\nEvents: Register", "State(s) in (\"\")"=w261, "State(s) at Back (\"\")"=w265) -> ("States Out"=w264:string)  [unwired: 12 in]
            n91 = call <vilib>:"Add State(s) to Queue__jki_lib_state_machine.vi"("State(s) in Front (\"\")"=w264, "State(s) in (\"\")"=w274) -> ("States Out"=w273:string)  [unwired: 13 in]
          }
          frame "Macro: Exit" {
            # "Exit Macro\n(This is called once, when the VI exits)"
            n92 = Unbundle By Name(w279) -> ("Core.Close Panel on Exit?"=w285:bool)
            n93 = Select(t="//UI: Front Panel State >> Closed", s=w285, f="") -> (s? t:f=w282:string)
            n94 = call <vilib>:"Add State(s) to Queue__jki_lib_state_machine.vi"("State(s) in Front (\"\")"="STP: Close\nData: Cleanup\nEvents: Unregister", "State(s) in (\"\")"="Process: Sync", "State(s) at Back (\"\")"="Exit") -> ("States Out"=w276:string)  [unwired: 12 in]
            n95 = call <vilib>:"Add State(s) to Queue__jki_lib_state_machine.vi"("State(s) in (\"\")"=w282, "State(s) at Back (\"\")"=w276) -> ("States Out"=w281:string)  [unwired: 13 in]
            n96 = call <vilib>:"Add State(s) to Queue__jki_lib_state_machine.vi"("State(s) in Front (\"\")"=w281, "State(s) in (\"\")"=w288) -> ("States Out"=w287:string)  [unwired: 13 in]
          }
          frame "---------- Process ----------" {
            # "Template Separator\n(You can make a copy of, or modify, this frame)"
            n97 = call <vilib>:"Add State(s) to Queue__jki_lib_state_machine.vi"("State(s) in (\"\")"=w293) -> ("States Out"=w292:string)  [unwired: 14 in]
          }
          frame "Process: Sync" {
            n98 = Unbundle By Name(w301) -> ("Self Reference"=w297:refnum<class "RemoteControl.lvclass">)
            n99 = call <vilib>:"WaitOnProcessSync.vi"("error in (no error)"=w296, "SMO"=w297) -> ("error out"=w295:errorcluster, "Don't run?"=w300:bool)  [unwired: 7 in, 1 out]
            n100 = Select(t="Data: Cleanup\nEvents: Unregister\nExit", s=w300, f="") -> (s? t:f=w294:string)
            n101 = call <vilib>:"Add State(s) to Queue__jki_lib_state_machine.vi"("State(s) in Front (\"\")"=w294, "State(s) in (\"\")"=w304) -> ("States Out"=w303:string)  [unwired: 13 in]
          }
          frame "---------- Events ----------" {
            # "Template Separator\n(You can make a copy of, or modify, this frame)"
            n102 = call <vilib>:"Add State(s) to Queue__jki_lib_state_machine.vi"("State(s) in (\"\")"=w309) -> ("States Out"=w308:string)  [unwired: 14 in]
          }
          frame "Events: Register" {
            # "Expand to add\nmore events"
            n103 = Unbundle By Name(w320) -> ("Self Reference"=w317:refnum<class "RemoteControl.lvclass">)
            n104 = call <vilib>:"GetProtectedEvents.vi"("SMO"=w317) -> ("error out"=w313:errorcluster, "SMO Protected Events"=w318:T28, "SMO out"=w312:refnum<class "RemoteControl.lvclass">)  [unwired: 8 in]
            n105 = call "RemoteControl.GetPrivateEvents.vi"("RemoteControl"=w312) -> ("error out"=w310:errorcluster, "Private Events"=w311:T29)  [unwired: 8 in, 1 out]
            n106 = register-events(w318, w311) -> (reference out=w319:refnum<event-registration>, error out=w314:errorcluster)  [unwired: 2 in]
            n107 = Merge Errors(w310, w316, w314, w313) -> (w315:errorcluster)
            n108 = call <vilib>:"Add State(s) to Queue__jki_lib_state_machine.vi"("State(s) in (\"\")"=w322) -> ("States Out"=w321:string)  [unwired: 14 in]
          }
          frame "Events: Unregister" {
            n109 = Unregister For Events(event registration refnum=w325, error in=w324) -> (error out=w323:errorcluster)
            n110 = call <vilib>:"Clear Errors.vi"("error in (no error)"=w323) -> ()  [unwired: 5 in, 2 out]
            n111 = call <vilib>:"Add State(s) to Queue__jki_lib_state_machine.vi"("State(s) in (\"\")"=w328) -> ("States Out"=w327:string)  [unwired: 14 in]
          }
          frame "---------- STP ----------" {
            n112 = call <vilib>:"Add State(s) to Queue__jki_lib_state_machine.vi"("State(s) in (\"\")"=w333) -> ("States Out"=w332:string)  [unwired: 14 in]
          }
          frame "STP: Wait Listener" {
            # "check here if remote\n= self or allowed"
            n113 = Unbundle By Name(w342) -> ("AllowedRemoteAddress"=w338:T8, "LocalAddress"=w339:string, "STP info.address"=w341:string, "STP info.port"=w340:u16)
            n114 = call <vilib>:"TCP Listen.vi"("error in (no error)"=w349, "timeout ms (wait forever: -1)"=100, "port"=w340, "service name"=w341) -> ("error out"=w344:errorcluster, "remote port"=w343:u16, "remote address"=w334:string, "connection ID"=w345:refnum<k5>)  [unwired: 3 in, 1 out]
            n115 = Equal?(x=w339, y=w334) -> (x = y?=w337:bool)
            n116 = Equal?(x=w338, y=w334) -> (x = y?=w336:bool)
            n117 = Or(x=w336, y=w337) -> (x .or. y?=w335:bool)
            n118 = case shown="No Error" w344 {
              selector: w344 -> [w355 w381]
              tunnel: w342 -> [w362 w378]
              tunnel: [w361 w378] -> w347
              tunnel: w345 -> [w360 _]
              tunnel: [w354 w380] -> w348
              tunnel: [w359 "" ("State(s) in Front (\"\")")] -> w346
              tunnel: w343 -> [w358 _]
              tunnel: w335 -> [w357 _]
              tunnel: w334 -> [w356 _]
              frame No Error {
                n119 = case shown="False" w357 {
                  tunnel: w362 -> [w367 w376]
                  tunnel: [w366 w375] -> w361
                  tunnel: w360 -> [w363 w374]
                  tunnel: w356 -> [w364 w373]
                  tunnel: ["STP: Close" ("State(s) in Front (\"\")") "STP: Write Commands" ("State(s) in Front (\"\")")] -> w359
                  tunnel: w358 -> [w365 w371]
                  tunnel: [w368 w370] -> w354
                  tunnel: w355 -> [w368 w370]
                  frame False {
                    n120 = Bundle By Name(cluster=w367, "STP info.STP connection info.connection ID"=w363, "remote address"=w364, "remote port"=w365) -> (w366:T25)
                  }
                  frame True {
                    n121 = Bundle By Name(cluster=w376, "STP info.STP connection info.connection ID"=w374, "remote address"=w373, "remote port"=w371) -> (w375:T25)
                  }
                }
              }
              frame Error {
                # "filter wait on listener timeout"
                n122 = call-poly <userlib>:"Filter Error Codes__ogtk.vi"("Error In"=w381, "Error Codes to Filter"=i32[] [56]) -> ("Error Out"=w380:errorcluster)  [unwired: 7 in, 2 out]
              }
            }
            n123 = call <vilib>:"Add State(s) to Queue__jki_lib_state_machine.vi"("State(s) in Front (\"\")"=w346, "State(s) in (\"\")"=w353) -> ("States Out"=w352:string)  [unwired: 13 in]
          }
          frame "STP: Write Commands" {
            n124 = Unbundle By Name(w388) -> ("STP info.STP connection info.meta data"=w382:T1[], "STP info.STP connection info.connection ID"=w386:refnum<k5>)
            n125 = call-poly <vilib>:"Write Meta Data.vi"("meta data"=w382, "error in"=w385, "connection ID"=w386) -> ("error out"=w384:errorcluster, "connection info out"=w383:T9)  [unwired: 7 in]
            n126 = Bundle By Name(cluster=w388, "STP info.STP connection info"=w383) -> (w387:T25)
            n127 = call <vilib>:"Add State(s) to Queue__jki_lib_state_machine.vi"("State(s) in (\"\")"=w391) -> ("States Out"=w390:string)  [unwired: 14 in]
          }
          frame "STP: Listen" {
            n128 = Unbundle By Name(w405) -> ("STP info.STP connection info"=w403:T9)
            n129 = call-poly <vilib>:"Read Message.vi"("options"=T7 {"ignore timeout error"=TRUE, "timeout ms (1000)"=1000}, "error in"=w402, "connection info in"=w403) -> ("error out"=w397:errorcluster, "name"=w398:T1, "data string"=w400:string, "connection info out"=w401:T9, "timed out?"=w392:bool)  [unwired: 3 in, 1 out]
            n130 = case shown="False" w392 {
              tunnel: w405 -> [w417 w431]
              tunnel: [w416 w431] -> w404
              tunnel: w401 -> [w414 _]
              tunnel: w400 -> [w413 _]
              tunnel: [w412 "STP: Close" ("States Out")] -> w399
              tunnel: w398 -> [w409 _]
              tunnel: w397 -> [w410 w433]
              tunnel: [w410 w432] -> w395
              frame False {
                n131 = String Length(string=w409) -> (length=w415:i32)
                n132 = call "StateHistory.vi"("Current State in"=w409) -> ("delimited string"=→"commands":string)  [unwired: 9 in, 1 out]
                n133 = case shown="\"ACK\"" w409 {
                  tunnel: w415 -> [_ _ w423]
                  tunnel: w413 -> [_ _ w422]
                  tunnel: ["STP: Close" ("State(s) in Front (\"\")") "STP: Acknowledge" ("State(s) in Front (\"\")") w421] -> w412
                  tunnel: w409 -> [_ _ w420]
                  frame "CLOSE" {
                  }
                  frame "ACK" {
                  }
                  frame "True", Default {
                    n134 = case shown="0" w423 {
                      tunnel: ["STP: Close" ("State with Arguments") w426] -> w421
                      tunnel: w420 -> [_ w428]
                      tunnel: w422 -> [_ _]
                      frame 0 {
                      }
                      frame 1, Default {
                        (unwired) "STP: Close" ("State(s) in Front (\"\")")
                        n135 = Concatenate Strings("Commands: " ("State(s) in Front (\"\")"), w428) -> (w429:string)
                        n136 = call <vilib>:"Build State String with Arguments__JKI_lib_State_Machine.vi"("State"=w429) -> ("State with Arguments"=w427:string)  [unwired: 5 in]
                        n137 = call <vilib>:"Add State(s) to Queue__jki_lib_state_machine.vi"("State(s) in Front (\"\")"=w427, "State(s) at Back (\"\")"="STP: Acknowledge" ("State(s) in Front (\"\")")) -> ("States Out"=w426:string)  [unwired: 13 in]
                      }
                    }
                  }
                }
                n138 = Bundle By Name(cluster=w417, "STP info.STP connection info"=w414, "data string"=w413, "command"=w409) -> (w416:T25)
                "command" <- w409
                "data string" <- w413
              }
              frame True {
                n139 = call <vilib>:"Clear Errors.vi"("error in (no error)"=w433) -> ("error out"=w432:errorcluster)  [unwired: 5 in, 1 out]
              }
            }
            n140 = call-poly <userlib>:"Filter Error Codes__ogtk.vi"("Error In"=w395, "Error Codes to Filter"=i32[] [1, 62, 64, 66]) -> ("Error Out"=w394:errorcluster)  [unwired: 7 in, 2 out]
            n141 = call <vilib>:"Add State(s) to Queue__jki_lib_state_machine.vi"("State(s) in Front (\"\")"=w399, "State(s) in (\"\")"=w408) -> ("States Out"=w407:string)  [unwired: 13 in]
          }
          frame "STP: Acknowledge" {
            n142 = local read "command"() -> (w435:T1)
            n143 = Unbundle By Name(w437) -> ("STP info.STP connection info"=w447:T9)
            n144 = Get Date/Time In Seconds() -> (seconds since 1Jan1904=w441:timestamp)
            n145 = Format Date/Time String(time format string (%c)="%H:%M:%S", seconds (now)=w441) -> (date/time string=w442:string)  [unwired: 1 in]
            n146 = Concatenate Strings(w435, " OK " ("data"), w442) -> (w439:string)
            n147 = call-poly <vilib>:"Write Message.vi"("error in"=w445, "data"=w439, "name"="ACK", "connection info in"=w447) -> ("error out"=w444:errorcluster, "connection info out"=w446:T9)  [unwired: 6 in]
            n148 = Bundle By Name(cluster=w437, "STP info.STP connection info"=w446) -> (w436:T25)
            n149 = call <vilib>:"Add State(s) to Queue__jki_lib_state_machine.vi"("State(s) in (\"\")"=w450) -> ("States Out"=w449:string)  [unwired: 14 in]
          }
          frame "STP: Unknown" {
            n150 = Unbundle By Name(w455) -> ("STP info.STP connection info"=w465:T9, "command"=w453:T1, "data string"=w452:string)
            n151 = Get Date/Time In Seconds() -> (seconds since 1Jan1904=w459:timestamp)
            n152 = Format Date/Time String(time format string (%c)="%H:%M:%S", seconds (now)=w459) -> (date/time string=w460:string)  [unwired: 1 in]
            n153 = call <vilib>:"Space Constant.vi"() -> ("String"=w451:string)
            n154 = Concatenate Strings(w453, w451, w452, " UNKNOWN " ("data"), w460) -> (w457:string)
            n155 = call-poly <vilib>:"Write Message.vi"("error in"=w463, "data"=w457, "name"="UNK", "connection info in"=w465) -> ("error out"=w462:errorcluster, "connection info out"=w464:T9)  [unwired: 6 in]
            n156 = Bundle By Name(cluster=w455, "STP info.STP connection info"=w464) -> (w454:T25)
            n157 = call <vilib>:"Add State(s) to Queue__jki_lib_state_machine.vi"("State(s) in (\"\")"=w468) -> ("States Out"=w467:string)  [unwired: 14 in]
          }
          frame "STP: Close" {
            n158 = Unbundle By Name(w472) -> ("STP info.STP connection info"=w473:T9)
            n159 = call-poly <vilib>:"Get Connection Reference.vi"("error in"=w475, "connection info in"=w473) -> ("error out"=w476:errorcluster, "connection ID out"=w477:refnum<k5>)  [unwired: 7 in, 1 out]
            n160 = TCP Close Connection(connection ID=w477, error in (no error)=w476) -> (error out=w474:errorcluster)  [unwired: 1 in, 1 out]
            n161 = call <vilib>:"Clear Errors.vi"("error in (no error)"=w474) -> ("error out"=w469:errorcluster)  [unwired: 5 in, 1 out]
            n162 = Bundle By Name(cluster=w472, "STP info.STP connection info.connection ID"=refnum<k5> refnum) -> (w471:T25)
            n163 = call <vilib>:"Add State(s) to Queue__jki_lib_state_machine.vi"("State(s) in (\"\")"=w480) -> ("States Out"=w479:string)  [unwired: 14 in]
          }
          frame "---------- Commands ----------" {
            n164 = call <vilib>:"Add State(s) to Queue__jki_lib_state_machine.vi"("State(s) in (\"\")"=w485) -> ("States Out"=w484:string)  [unwired: 14 in]
          }
          frame "Commands: configAO" {
            w488 = T30 {"Channels: AO"={"AO amp (V)"=[0.01, 0.0, 0.0, 0.0, 0.0, 0.0, 0.0, 0.0], "AO DC (V)"=[0.0, 0.0, 0.0, 0.0, 0.0, 0.0, 0.0, 0.0], "AO f (Hz)"=[13.1, 13.0, 13.0, 13.0, 13.0, 13.0, 13.0, 13.0], "AO phi (deg)"=[0.0, 0.0, 0.0, 0.0, 0.0, 0.0, 0.0, 0.0], "function"=[enum."Sine Wave", enum."Sine Wave", enum."Sine Wave", enum."Sine Wave", enum."Sine Wave", enum."Sine Wave", enum."Sine Wave", enum."Sine Wave"]}} ("configAO")
            n165 = Unbundle By Name(w493) -> ("Self Reference"=w497:refnum<class "RemoteControl.lvclass">, "data string"=w494:string)
            n166 = Unbundle By Name(w488) -> ("Channels: AO"=w486:T14)
            n167 = call <vilib>:"Unflatten From JSON String.vi"("Type and Defaults"=w486, "error in (no error)"=w492, "JSON String"=w494) -> ("error out"=w495:errorcluster, "Variant"=w496:variant)  [unwired: 7 in]
            n168 = Variant To Data(error in=w495, type=w486, Variant=w496) -> (data=w487:T14, error out=w490:errorcluster)
            n169 = Bundle By Name(cluster=w488, "Channels: AO"=w487) -> (w489:T30)
            n170 = call "RemoteControl.configAO.vi"("error in (no error)"=w490, "configAO"=w489, "RemoteControl"=w497) -> ("error out"=w491:errorcluster)  [unwired: 7 in, 1 out]
            n171 = call <vilib>:"Add State(s) to Queue__jki_lib_state_machine.vi"("State(s) in (\"\")"=w500) -> ("States Out"=w499:string)  [unwired: 14 in]
          }
          frame "Commands: configREF" {
            w504 = T31 {"Channels: Lockin"={"REF f (Hz)"=[13.0], "REF phi (deg)"=[0.0, 0.0, 0.0, 0.0, 0.0, 0.0, 0.0, 0.0]}} ("configREF")
            n172 = Unbundle By Name(w507) -> ("Self Reference"=w508:refnum<class "RemoteControl.lvclass">, "data string"=w511:string)
            n173 = Unbundle By Name(w504) -> ("Channels: Lockin"=w503:T21)
            n174 = call <vilib>:"Unflatten From JSON String.vi"("Type and Defaults"=w503, "error in (no error)"=w506, "JSON String"=w511) -> ("error out"=w510:errorcluster, "Variant"=w509:variant)  [unwired: 7 in]
            n175 = Variant To Data(error in=w510, type=w503, Variant=w509) -> (data=w502:T21, error out=w512:errorcluster)
            n176 = Bundle By Name(cluster=w504, "Channels: Lockin"=w502) -> (w501:T31)
            n177 = call "RemoteControl.configREF.vi"("error in (no error)"=w512, "configREF"=w501, "RemoteControl"=w508) -> ("error out"=w505:errorcluster)  [unwired: 7 in, 1 out]
            n178 = call <vilib>:"Add State(s) to Queue__jki_lib_state_machine.vi"("State(s) in (\"\")"=w515) -> ("States Out"=w514:string)  [unwired: 14 in]
          }
          frame "Commands: configIVmode" {
            w522 = T32 TRUE  # configIVmode
            n179 = Unbundle By Name(w516) -> ("Self Reference"=w525:refnum<class "RemoteControl.lvclass">, "data string"=w519:string)
            n180 = call <vilib>:"Unflatten From JSON String.vi"("Type and Defaults"=w522, "error in (no error)"=w520, "JSON String"=w519) -> ("error out"=w523:errorcluster, "Variant"=w524:variant)  [unwired: 7 in]
            n181 = Variant To Data(error in=w523, type=w522, Variant=w524) -> (data=w521:T32, error out=w518:errorcluster)
            n182 = call "RemoteControl.configIVmode.vi"("error in (no error)"=w518, "configIVmode"=w521, "RemoteControl"=w525) -> ("error out"=w517:errorcluster)  [unwired: 7 in, 1 out]
            n183 = call <vilib>:"Add State(s) to Queue__jki_lib_state_machine.vi"("State(s) in (\"\")"=w528) -> ("States Out"=w527:string)  [unwired: 14 in]
          }
          frame "Commands: configRemote" {
            w529 = T33 TRUE  # configRemote
            n184 = Unbundle By Name(w537) -> ("Self Reference"=w538:refnum<class "RemoteControl.lvclass">, "data string"=w532:string)
            n185 = call <vilib>:"Unflatten From JSON String.vi"("Type and Defaults"=w529, "error in (no error)"=w533, "JSON String"=w532) -> ("error out"=w534:errorcluster, "Variant"=w535:variant)  [unwired: 7 in]
            n186 = Variant To Data(error in=w534, type=w529, Variant=w535) -> (data=w531:T33, error out=w530:errorcluster)
            n187 = call "RemoteControl.configRemote.vi"("error in (no error)"=w530, "configRemote"=w531, "RemoteControl"=w538) -> ("error out"=w536:errorcluster)  [unwired: 7 in, 1 out]
            n188 = call <vilib>:"Add State(s) to Queue__jki_lib_state_machine.vi"("State(s) in (\"\")"=w541) -> ("States Out"=w540:string)  [unwired: 14 in]
          }
          frame "Commands: configReset" {
            w546 = T34 FALSE ("configReset")
            n189 = Unbundle By Name(w551) -> ("Self Reference"=w545:refnum<class "RemoteControl.lvclass">, "data string"=w547:string)
            n190 = call <vilib>:"Unflatten From JSON String.vi"("Type and Defaults"=w546, "error in (no error)"=w548, "JSON String"=w547) -> ("error out"=w549:errorcluster, "Variant"=w550:variant)  [unwired: 7 in]
            n191 = Variant To Data(error in=w549, type=w546, Variant=w550) -> (data=w544:T34, error out=w542:errorcluster)
            n192 = call "RemoteControl.configReset.vi"("error in (no error)"=w542, "configReset"=w544, "RemoteControl"=w545) -> ("error out"=w543:errorcluster)  [unwired: 7 in, 1 out]
            n193 = call <vilib>:"Add State(s) to Queue__jki_lib_state_machine.vi"("State(s) in (\"\")"=w554) -> ("States Out"=w553:string)  [unwired: 14 in]
          }
          frame "Commands: assertTrigger" {
            w559 = T35 FALSE  # assertTrigger
            n194 = Unbundle By Name(w564) -> ("Self Reference"=w558:refnum<class "RemoteControl.lvclass">, "data string"=w560:string)
            n195 = call <vilib>:"Unflatten From JSON String.vi"("Type and Defaults"=w559, "error in (no error)"=w561, "JSON String"=w560) -> ("error out"=w562:errorcluster, "Variant"=w563:variant)  [unwired: 7 in]
            n196 = Variant To Data(error in=w562, type=w559, Variant=w563) -> (data=w557:T35, error out=w556:errorcluster)
            n197 = call "RemoteControl.assertTrigger.vi"("error in (no error)"=w556, "assertTrigger"=w557, "RemoteControl"=w558) -> ("error out"=w555:errorcluster)  [unwired: 7 in, 1 out]
            n198 = call <vilib>:"Add State(s) to Queue__jki_lib_state_machine.vi"("State(s) in (\"\")"=w567) -> ("States Out"=w566:string)  [unwired: 14 in]
          }
          frame "Commands: getAO" {
            n199 = Unbundle By Name(w576) -> ("STP info.STP connection info"=w572:T9, "command"=w573:T1, "setAO"=w568:T10)
            n200 = Flatten To String(anything=w568, prepend array or string size? (T)=TRUE ("Multiline (T)"), error in (no error)=w571) -> (data string=w575:string, error out=w574:errorcluster)  [unwired: 1 in, 1 out]
            n201 = call-poly <vilib>:"Write Message.vi"("error in"=w574, "data"=w575, "name"=w573, "connection info in"=w572) -> ("error out"=w570:errorcluster)  [unwired: 6 in, 1 out]
            n202 = call <vilib>:"Add State(s) to Queue__jki_lib_state_machine.vi"("State(s) in (\"\")"=w579) -> ("States Out"=w578:string)  [unwired: 14 in]
          }
          frame "Commands: getAI" {
            n203 = Unbundle By Name(w587) -> ("STP info.STP connection info"=w583:T9, "command"=w584:T1, "setAI"=w588:T11)
            n204 = Flatten To String(anything=w588, prepend array or string size? (T)=TRUE ("Multiline (T)"), error in (no error)=w582) -> (data string=w586:string, error out=w585:errorcluster)  [unwired: 1 in, 1 out]
            n205 = call-poly <vilib>:"Write Message.vi"("error in"=w585, "data"=w586, "name"=w584, "connection info in"=w583) -> ("error out"=w581:errorcluster)  [unwired: 6 in, 1 out]
            n206 = call <vilib>:"Add State(s) to Queue__jki_lib_state_machine.vi"("State(s) in (\"\")"=w591) -> ("States Out"=w590:string)  [unwired: 14 in]
          }
          frame "Commands: getResults" {
            n207 = Unbundle By Name(w599) -> ("STP info.STP connection info"=w595:T9, "command"=w596:T1, "setResults"=w600:T12)
            n208 = Flatten To String(anything=w600, prepend array or string size? (T)=TRUE ("Multiline (T)"), error in (no error)=w594) -> (data string=w598:string, error out=w597:errorcluster)  [unwired: 1 in, 1 out]
            n209 = call-poly <vilib>:"Write Message.vi"("error in"=w597, "data"=w598, "name"=w596, "connection info in"=w595) -> ("error out"=w593:errorcluster)  [unwired: 6 in, 1 out]
            n210 = call <vilib>:"Add State(s) to Queue__jki_lib_state_machine.vi"("State(s) in (\"\")"=w603) -> ("States Out"=w602:string)  [unwired: 14 in]
          }
          frame "Commands: getTrigger" {
            n211 = Unbundle By Name(w611) -> ("STP info.STP connection info"=w607:T9, "command"=w608:T1, "setTrigger"=w612:T13)
            n212 = Flatten To String(anything=w612, prepend array or string size? (T)=TRUE ("Multiline (T)"), error in (no error)=w606) -> (data string=w610:string, error out=w609:errorcluster)  [unwired: 1 in, 1 out]
            n213 = call-poly <vilib>:"Write Message.vi"("error in"=w609, "data"=w610, "name"=w608, "connection info in"=w607) -> ("error out"=w605:errorcluster)  [unwired: 6 in, 1 out]
            n214 = call <vilib>:"Add State(s) to Queue__jki_lib_state_machine.vi"("State(s) in (\"\")"=w615) -> ("States Out"=w614:string)  [unwired: 14 in]
          }
          frame "Commands: getIVmode" {
            n215 = Unbundle By Name(w623) -> ("STP info.STP connection info"=w619:T9, "command"=w620:T1, "setIVmode"=w624:T24)
            n216 = Flatten To String(anything=w624, prepend array or string size? (T)=TRUE ("Multiline (T)"), error in (no error)=w618) -> (data string=w622:string, error out=w621:errorcluster)  [unwired: 1 in, 1 out]
            n217 = call-poly <vilib>:"Write Message.vi"("error in"=w621, "data"=w622, "name"=w620, "connection info in"=w619) -> ("error out"=w617:errorcluster)  [unwired: 6 in, 1 out]
            n218 = call <vilib>:"Add State(s) to Queue__jki_lib_state_machine.vi"("State(s) in (\"\")"=w627) -> ("States Out"=w626:string)  [unwired: 14 in]
          }
          frame "Commands: getAOconfig" {
            n219 = Unbundle By Name(w635) -> ("STP info.STP connection info"=w631:T9, "command"=w632:T1, "Channels: AO"=w636:T14)
            n220 = Flatten To String(anything=w636, prepend array or string size? (T)=TRUE ("Multiline (T)"), error in (no error)=w630) -> (data string=w634:string, error out=w633:errorcluster)  [unwired: 1 in, 1 out]
            n221 = call-poly <vilib>:"Write Message.vi"("error in"=w633, "data"=w634, "name"=w632, "connection info in"=w631) -> ("error out"=w629:errorcluster)  [unwired: 6 in, 1 out]
            n222 = call <vilib>:"Add State(s) to Queue__jki_lib_state_machine.vi"("State(s) in (\"\")"=w639) -> ("States Out"=w638:string)  [unwired: 14 in]
          }
          frame "Commands: getREFconfig" {
            n223 = Unbundle By Name(w647) -> ("STP info.STP connection info"=w643:T9, "command"=w644:T1, "Channels: Lockin"=w648:T21)
            n224 = Flatten To String(anything=w648, prepend array or string size? (T)=TRUE ("Multiline (T)"), error in (no error)=w642) -> (data string=w646:string, error out=w645:errorcluster)  [unwired: 1 in, 1 out]
            n225 = call-poly <vilib>:"Write Message.vi"("error in"=w645, "data"=w646, "name"=w644, "connection info in"=w643) -> ("error out"=w641:errorcluster)  [unwired: 6 in, 1 out]
            n226 = call <vilib>:"Add State(s) to Queue__jki_lib_state_machine.vi"("State(s) in (\"\")"=w651) -> ("States Out"=w650:string)  [unwired: 14 in]
          }
        }
      }
    }
    frame Error {
    }
  }
  n227 = call-parent "Process.vi"("error in"=w7, "SMO"=w6) -> ("error out"=w4:errorcluster, "SMO out"=→"RemoteControl out":refnum<class "RemoteControl.lvclass">)  [unwired: 8 in]
  n228 = Merge Errors(w4, w3) -> (→"error out":errorcluster)
